vi "Measurement Logic.vi"(8 "error in":errorcluster, 9 "measurement configuration":T2={"Capturing Stream"=TRUE, "Pause Capture"=FALSE, "Interface Name"="Lorem ipsum dolor sit"}, 10 "measure call context in":refnum<class "Measure Call Context.lvclass">) -> (0 "error out":errorcluster, 1 "measurement results":T1, 2 "measure call context out":refnum<class "Measure Call Context.lvclass">)   [LabVIEW 2025, in "Automotive Ethernet Bus Monitor.lvclass"]
doc: "Contains the core logic for executing the measurement."
uses:
  Automotive Ethernet Bus Monitor.lvclass
  Automotive Ethernet Bus Monitor.lvclass/Automotive Ethernet Bus Monitor.ctl
  Measurement Results.ctl
  <vilib>/xnet/xnet.llb/XNET Create Session (Frame Input Stream).vi
  <vilib>/xnet/xnet.llb/XNET Read (Frame Ethernet).vi
  <resource>/objmgr/xnet.rc
  <vilib>/Plug-In SDKs/Measurements/Measure Call Context/Measure Call Context.lvclass
  Measurement Configuration.ctl
panel:
  in  "Packets":i32
  out "interface open":bool=TRUE
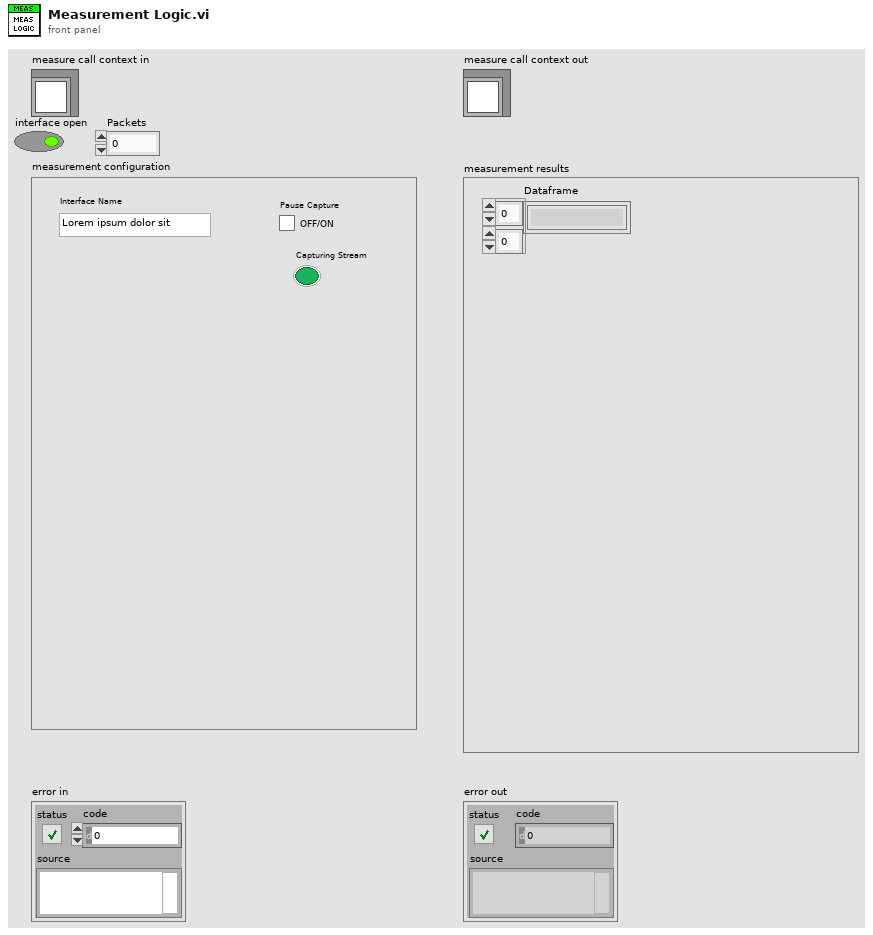
[diagram p1: front panel]
types:
  T1 = typedef "Automotive Ethernet Bus Monitor.lvclass/Measurement Results.ctl" = cluster{"Dataframe":string[][]}
  T2 = typedef "Automotive Ethernet Bus Monitor.lvclass/Measurement Configuration.ctl" = cluster{"Capturing Stream":bool, "Pause Capture":bool, "Interface Name":string}
  T3 = typedef "XNET Frame Ethernet.ctl" = cluster{"local timestamp":timestamp, "network timestamp":timestamp, "frame data":u8[], "fcs":u32, "type":T4, "network synced?":bool, "receive?":bool, "transmit?":bool, "error?":bool}
  T4 = typedef "XNET Frame Type Ethernet.ctl" = u16
  T5 = typedef "Event Messenger-bool.lvlib/))Channel.ctl" = refnum<queue>
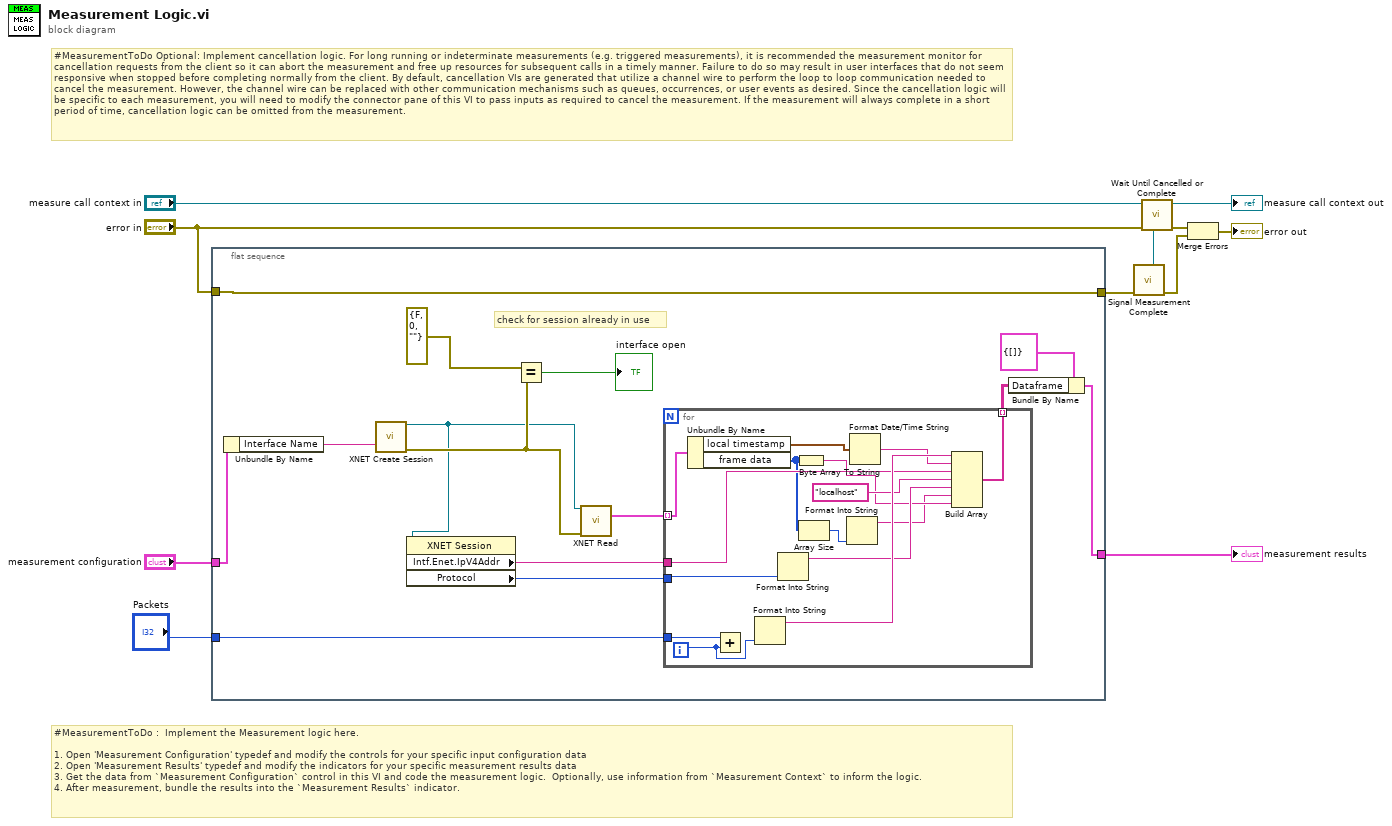
[diagram p0: block diagram]
diagram:
  # "#MeasurementToDo Optional: Implement cancellation logic. For long running or indeterminate measurements (e.g. triggered measurements), it is recommended the measurement monitor for cancellation requests from the client so it can abort the measurement and free up resources for subsequent calls in a timely manner. Failure to do so may result in user interfaces that do not seem responsive when stopped before completing normally from the client. By default, cancellation VIs are generated that utilize a channel wire to perform the loop to loop communication needed to cancel the measurement. However, the channel wire can be replaced with other communication mechanisms such as queues, occurrences, or user events as desired. Since the cancellation logic will be specific to each measurement, you will need to modify the connector pane of this VI to pass inputs as required to cancel the measurement. If the measurement will always complete in a short period of time, cancellation logic can be omitted from the measurement."
  # "#MeasurementToDo :  Implement the Measurement logic here.\n\n1. Open 'Measurement Configuration' typedef and modify the controls for your specific input configuration data\n2. Open 'Measurement Results' typedef and modify the indicators for your specific measurement results data\n3. Get the data from `Measurement Configuration` control in this VI and code the measurement logic.  Optionally, use information from `Measurement Context` to inform the logic.\n4. After measurement, bundle the results into the `Measurement Results` indicator."
  n1 = flat-sequence {
    tunnel: "measurement configuration" -> [w24]
    tunnel: "error in" -> [w25]
    tunnel: [w25] -> w7
    tunnel: "Packets" -> [w17]
    tunnel: [w12] -> w1
    frame #0 {
      # "check for session already in use"
      n2 = Unbundle By Name(w24) -> ("Interface Name"=w23:string)
      n3 = call-poly <vilib>:"XNET Create Session.vi"("interface"=w23) -> ("session out"=w18:refnum<k21>, "error out"=w20:errorcluster)  [unwired: 13 in]
      n4 = property class="XNET Session"(reference=w18) -> ("Intf.Enet.IpV4Addr"=w16:string, "Protocol"=w15:u32)  [unwired: 1 in, 2 out]
      n5 = Equal?(x=errorcluster {"status"=FALSE, "code"=0, "source"=""}, y=w20) -> (x = y?=→"interface open":bool)
      n6 = call-poly <vilib>:"XNET Read.vi"("session in"=w18, "error in (no error)"=w20) -> ("data"=w19:T3[])  [unwired: 10 in, 3 out]
      n7 = for {
        tunnel: w19 -> [w40] mode=indexing
        tunnel: w17 -> [w39]
        tunnel: w16 -> [w34]
        tunnel: w15 -> [w32]
        tunnel: [w26] -> w13 mode=indexing
        i -> [w38]
        n8 = Unbundle By Name(w40) -> ("local timestamp"=w36:timestamp, "frame data"=w29:u8[])
        n9 = Add(x=w39, y=w38) -> ()  [unwired: 1 out]
        n10 = Format Into String(w38) -> (resulting string=w37:string)  [unwired: 3 in, 1 out]
        n11 = Format Into String(w32) -> (resulting string=w31:string)  [unwired: 3 in, 1 out]
        n12 = Byte Array To String(unsigned byte array=w29) -> (string=w30:string)
        n13 = Array Size(array=w29) -> (size(s)=w28:i32)
        n14 = Format Into String(w28) -> (resulting string=w27:string)  [unwired: 3 in, 1 out]
        n15 = Format Date/Time String(seconds (now)=w36) -> (date/time string=w35:string)  [unwired: 2 in]
        n16 = Build Array(w37, w35, w34, "localhost" ("element"), w31, w27, w30) -> (w26:string[])
      }
      n17 = Bundle By Name(cluster=T1 {"Dataframe"=[]} ("Measurement Results"), "Dataframe"=w13) -> (w12:T1)
    }
  }
  n18 = call "Signal Measurement Complete.vi"("error in (no error)"=w7) -> ("error out"=w5:errorcluster, "done channel"=w6:T5)  [unwired: 9 in]
  n19 = call "Wait Until Cancelled or Complete.vi"("done channel"=w6, "error in (no error)"="error in", "measure call context in"="measure call context in") -> ("error out"=w4:errorcluster, "measure call context out"=→"measure call context out":refnum<class "Measure Call Context.lvclass">)  [unwired: 7 in]
  n20 = Merge Errors(w4, w5) -> (→"error out":errorcluster)
  "measurement results" <- w1
